vi "Teleop.vi"(10 "Match Info":T2={"Autonomous Elapsed Seconds"=0.0, "TeleOp Elapsed Seconds"=0.0, "Disabled Elapsed Seconds"=0.0, "Visited Autonomous"=FALSE, "Visited TeleOp"=FALSE, "Visited Disabled"=FALSE, "Autonomous Settings"={"Autonomous Style"=enum."Independent", "VI Refnum"=refnum}}, 11 "Call Context":T3) -> ()   [LabVIEW 2019]
doc: "This VI is called for each TeleOp packet received from the DS where the robot is not disabled. It is often used to read from the joysticks and update I/O or to update setpoints for timed control loops. It should complete and return within 20 milliseconds or it may miss DS packets."
uses:
  <vilib>/Rock Robotics/WPI/DriverStation/WPI_DriverStationDerivedRobotMode.ctl
  <vilib>/Rock Robotics/WPI/DriverStation/WPI_DriverStationMatch Info.ctl
  <vilib>/Rock Robotics/WPI/Utilities/WPI_GetSetVariantRefNum.vi
  <vilib>/Rock Robotics/Network Tables/NT Write Boolean Array.vi
  <vilib>/Rock Robotics/Network Tables/NT Write Numeric Array.vi
  <vilib>/Rock Robotics/Network Tables/NT Read Boolean.vi
  <vilib>/Rock Robotics/Network Tables/NT Read Number.vi
  <vilib>/Rock Robotics/Network Tables/NT Write Number.vi
  <vilib>/Rock Robotics/WPI/RobotDrive/WPI_RobotDriveMecanumDrive_Cartesian.vi
  <vilib>/Instr/_visa.llb/VISA Configure Serial Port (Instr).vi
  <vilib>/Rock Robotics/Network Tables/NT Write String.vi
panel:
  out "read buffer":string="0"
  out "return count":u32
  out "Continuous Angle":T1
  out "x":i16
  out "Matched Color Name":string
  out "Match Confidence":dbl
  out "Measured Color":cluster{"R":dbl, "G":dbl, "B":dbl}
  out "error out":errorcluster
  out "Color":u32(colorbox)
  in  "Blue Calibration":cluster{"R":dbl, "G":dbl, "B":dbl}={"R"=0.143, "G"=0.427, "B"=0.429}
  in  "Green Calibration":cluster{"R":dbl, "G":dbl, "B":dbl}={"R"=0.197, "G"=0.561, "B"=0.24}
  in  "Red Calibration":cluster{"R":dbl, "G":dbl, "B":dbl}={"R"=0.561, "G"=0.323, "B"=0.114}
  in  "Yellow Calibration":cluster{"R":dbl, "G":dbl, "B":dbl}={"R"=0.361, "G"=0.524, "B"=0.113}
  out "Elapsed Time Since Reset (s)":i32 caption="Elapsed Time (s)"
  out "Sample Slider 0":dbl(slide) scale=0.0..5.0
  out "Sample Boolean 1":bool
  out "Sample Boolean 0":bool
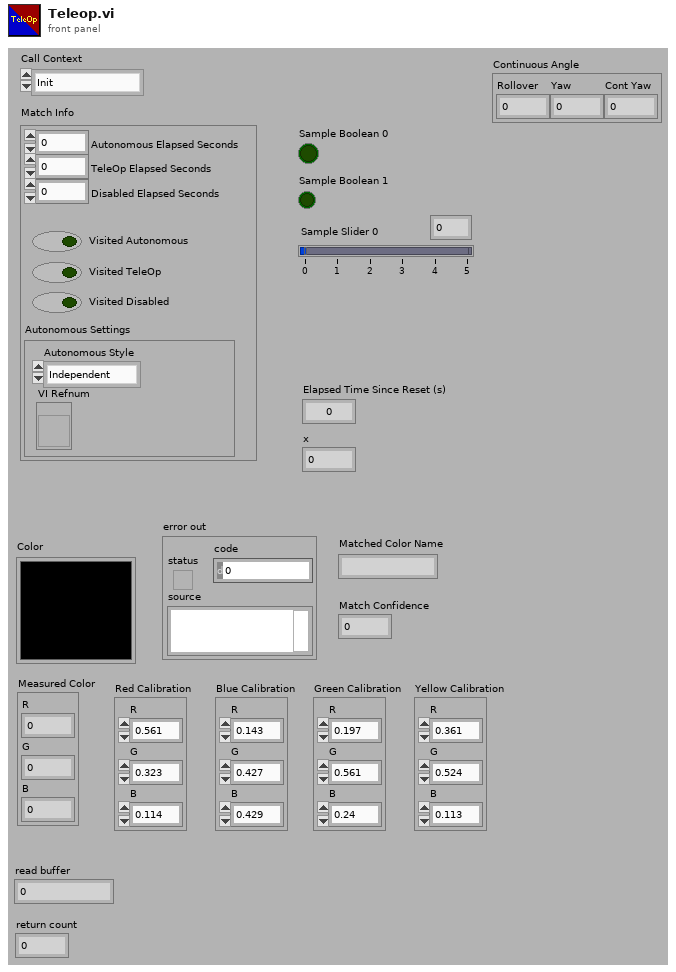
[diagram p1: front panel]
types:
  T1 = cluster{"Rollover":dbl, "Yaw":dbl, "Cont Yaw":dbl}
  T2 = typedef "WPI_DriverStationMatch Info.ctl" = cluster{"Autonomous Elapsed Seconds":dbl, "TeleOp Elapsed Seconds":dbl, "Disabled Elapsed Seconds":dbl, "Visited Autonomous":bool, "Visited TeleOp":bool, "Visited Disabled":bool, "Autonomous Settings":cluster{"Autonomous Style":enum16{"Iterative", "Independent"}, "VI Refnum":refnum<vi>}}
  T3 = typedef "WPI_DriverStationDerivedRobotMode.ctl" = enum16{"Init", "Execute", "Stop"}
  T4 = typedef "Color Sensor V3 DevRef.ctl" = cluster{"I2CDevRef":T5}
  T5 = typedef "WPI_I2CDevRef.ctl" = cluster{"DevStatus":errorcluster, "Device Address":u8, "Handle":i32, "I2C Bus":T6}
  T6 = typedef "i2c_bus.ctl" = enum16{"I2C On-Board", "I2C MXP", "Invalid"}
  T7 = typedef "WPI_RobotDriveDevRef.ctl" = cluster{"DevStatus":errorcluster, "Motors[]":T8[], "Square Inputs":bool, "Max Output":dbl}
  T8 = typedef "WPI_MotorControlDeviceRef.ctl" = cluster{"DeviceStatus":errorcluster, "Type":T9, "PWM":cluster{"PWM Channel":T10, "DeadBand":T11}, "CAN":cluster{"Device Number":u8, "SetOutput VI Ref":variant, "GetOutput VI Ref":variant, "Enable VI Ref":variant, "Disable VI Ref":variant, "Data":variant}, "Invert":bool, "DIO PWM":cluster{"PWM \"Enable\" Channel":T10, "DIOChannel":T12, "PWM Rate":dbl}}
  T9 = typedef "WPI_MotorControlType.ctl" = enum16{"PWM", "CAN", "DIO PWM"}
  T10 = typedef "FPGA_DIOPWMChannel.ctl" = enum8{"PWM 0", "PWM 1", "PWM 2", "PWM 3", "PWM 4", "PWM 5", "PWM 6", "PWM 7", "PWM 8", "PWM 9", "PWM MXP 0", "PWM MXP 1", "PWM MXP 2", "PWM MXP 3", "PWM MXP 4", "PWM MXP 5", "PWM MXP 6", "PWM MXP 7", "PWM MXP 8", "PWM MXP 9", "Invalid"}
  T11 = typedef "WPI_PWMDeadband.ctl" = cluster{"Name":string, "maxPositivePwm":i32, "minPositivePwm":i32, "centerPwm":i32, "maxNegativePwm":i32, "minNegativePwm":i32, "angularRange":u16}
  T12 = typedef "FPGA_DIOChannel.ctl" = enum8{"DIO 0", "DIO 1", "DIO 2", "DIO 3", "DIO 4", "DIO 5", "DIO 6", "DIO 7", "DIO 8", "DIO 9", "DIO MXP 0", "DIO MXP 1", "DIO MXP 2", "DIO MXP 3", "DIO MXP 4", "DIO MXP 5", "DIO MXP 6", "DIO MXP 7", "DIO MXP 8", "DIO MXP 9", "DIO MXP 10", "DIO MXP 11", "DIO MXP 12", "DIO MXP 13", "DIO MXP 14", "DIO MXP 15", "SPI Port CS1", "SPI Port CS2", "SPI Port CS3", "SPI Port MISO", "SPI Port MOSI", "Invalid"}
  T13 = typedef "WPI_JoystickDevRef.ctl" = cluster{"Device":T14}
  T14 = typedef "WPI_JoystickDeviceEnum.ctl" = enum16{"USB 0", "USB 1", "USB 2", "USB 3", "USB 4", "USB 5"}
  T15 = typedef "WPI_SwitchDevRef.ctl" = cluster{"DevStatus":errorcluster, "DIO Channel":T12, "CntIndex":T16, "Normally Closed":bool}
  T16 = typedef "FPGA_CounterCtrSystemIndex.ctl" = enum8{"Ctr 0", "Ctr 1", "Ctr 2", "Ctr 3", "Ctr 4", "Ctr 5", "Ctr 6", "Ctr 7", "Invalid"}
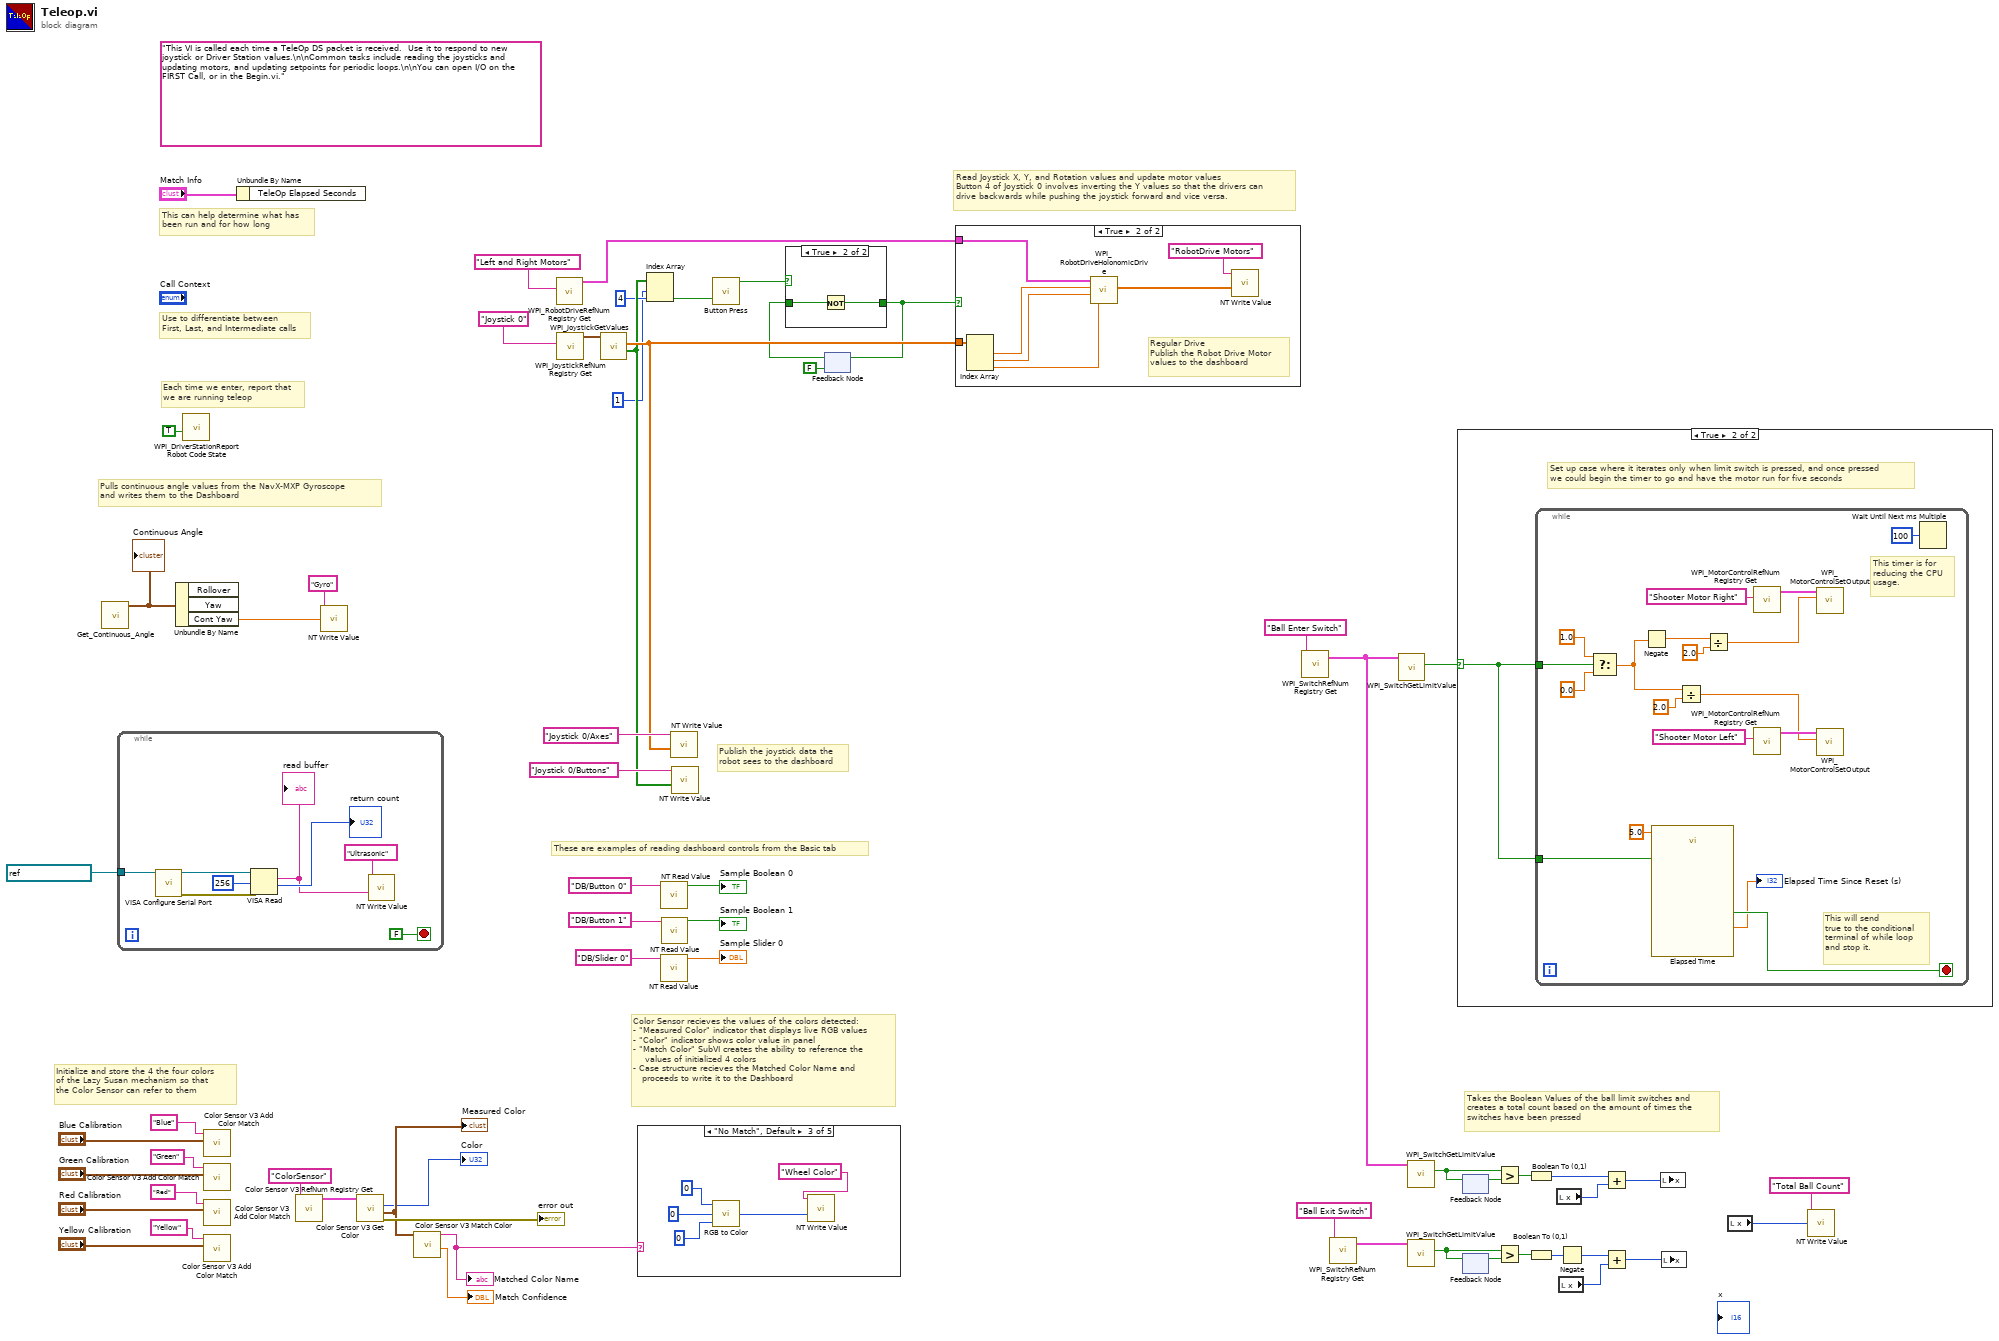
[diagram p0: block diagram]
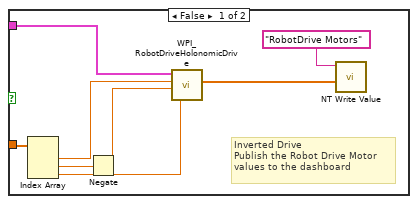
[diagram p2: hidden frame]
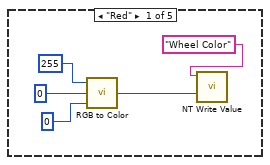
[diagram p4: hidden frame]
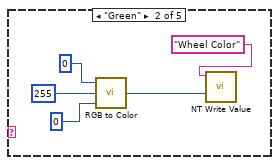
[diagram p5: hidden frame]
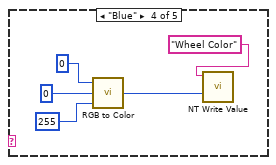
[diagram p6: hidden frame]
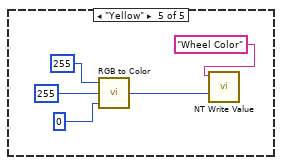
[diagram p7: hidden frame]
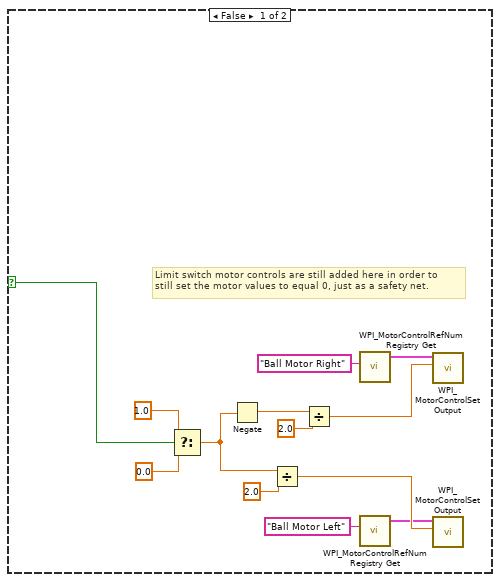
[diagram p8: hidden frame]
diagram:
  (unwired) "This VI is called each time a TeleOp DS packet is received.  Use it to respond to new joystick or Driver Station values.\n\nCommon tasks include reading the joysticks and updating motors, and updating setpoints for periodic loops.\n\nYou can open I/O on the FIRST Call, or in the Begin.vi."
  # "Takes the Boolean Values of the ball limit switches and \ncreates a total count based on the amount of times the \nswitches have been pressed"
  # "Pulls continuous angle values from the NavX-MXP Gyroscope\nand writes them to the Dashboard"
  # "Color Sensor recieves the values of the colors detected:\n- \"Measured Color\" indicator that displays live RGB values\n- \"Color\" indicator shows color value in panel\n- \"Match Color\" SubVI creates the ability to reference the \n    values of initialized 4 colors\n- Case structure recieves the Matched Color Name and \n   proceeds to write it to the Dashboard"
  # "Initialize and store the 4 the four colors \nof the Lazy Susan mechanism so that \nthe Color Sensor can refer to them"
  # "These are examples of reading dashboard controls from the Basic tab"
  # "Publish the joystick data the\nrobot sees to the dashboard"
  # "Each time we enter, report that\nwe are running teleop"
  # "Use to differentiate between\nFirst, Last, and Intermediate calls"
  # "This can help determine what has\nbeen run and for how long"
  # "Read Joystick X, Y, and Rotation values and update motor values\nButton 4 of Joystick 0 involves inverting the Y values so that the drivers can\ndrive backwards while pushing the joystick forward and vice versa."
  n1 = call <vilib>:"Get_Continuous_Angle.vi"() -> ("Continuous Angle"=w2:T1)  [unwired: 11 in]
  "Continuous Angle" <- w2
  n2 = while {
    tunnel: refnum<visa-resource-name> "ASRL3::INSTR" ("VISA resource name") -> [w66]
    stop <- FALSE stop-if-true
    n3 = call-poly "VISA Configure Serial Port"("VISA resource name"=w66) -> ("VISA resource name out"=w70:refnum<visa-resource-name>, "error out"=w68:errorcluster)  [unwired: 13 in]
    n4 = VISA Read(VISA resource name=w70, byte count=u32 256, error in (no error)=w68) -> (read buffer=w63:string, return count=→"return count":u32)  [unwired: 2 out]
    "read buffer" <- w63
    n5 = call-poly <vilib>:"NT Write Value.vi"("String"=w63, "Name"="Ultrasonic") -> ()  [unwired: 9 in, 1 out]
  }
  n6 = Unbundle By Name(w2) -> ("Cont Yaw"=w4:dbl)  [unwired: 2 out]
  n7 = call <vilib>:"WPI_DriverStationReport Robot Code State.vi"("TeleOp"=TRUE ("Autonomous")) -> ()  [unwired: 10 in, 1 out]
  n8 = call <vilib>:"Color Sensor V3 Add Color Match.vi"("Color"="Blue Calibration", "Name"="Blue") -> ()  [unwired: 10 in]
  n9 = call <vilib>:"Color Sensor V3 Add Color Match.vi"("Color"="Green Calibration", "Name"="Green") -> ()  [unwired: 10 in]
  n10 = call <vilib>:"Color Sensor V3 Add Color Match.vi"("Color"="Red Calibration", "Name"="Red") -> ()  [unwired: 10 in]
  n11 = call <vilib>:"Color Sensor V3 Add Color Match.vi"("Color"="Yellow Calibration", "Name"="Yellow") -> ()  [unwired: 10 in]
  n12 = Unbundle By Name("Match Info") -> ()  [unwired: 1 out]
  n13 = call <vilib>:"Color Sensor V3 RefNum Registry Get.vi"("refnum name"="ColorSensor") -> ("ColorSensorDevRef"=w32:T4)  [unwired: 9 in, 1 out]
  n14 = call-poly <vilib>:"NT Write Value.vi"("Numeric"=w4, "Name"="Gyro") -> ()  [unwired: 9 in, 1 out]
  n15 = call <vilib>:"Color Sensor V3 Get Color.vi"("ColorSensorDevRef"=w32) -> ("error out"=→"error out":errorcluster, "Normalized Color"=w34:cluster{"R":dbl, "G":dbl, "B":dbl}, "Color"=→"Color":u32)  [unwired: 7 in, 1 out]
  "Measured Color" <- w34
  n16 = call <vilib>:"Color Sensor V3 Match Color.vi"("Measured Color"=w34) -> ("Confidence"=→"Match Confidence":dbl, "Matched Color Name"=w21:string)  [unwired: 8 in, 1 out]
  "Matched Color Name" <- w21
  n17 = call <vilib>:"WPI_RobotDriveRefNum Registry Get.vi"("refnum name"="Left and Right Motors") -> ("RobotDriveDevRef"=w22:T7)  [unwired: 1 in, 9 out]
  n18 = call <vilib>:"WPI_JoystickRefNum Registry Get.vi"("refnum name"="Joystick 0") -> ("JoystickDevRef"=w59:T13)  [unwired: 1 in, 9 out]
  n19 = call <vilib>:"WPI_JoystickGetValues.vi"("JoystickDevRef"=w59) -> ("Buttons"=w20:bool[], "Axes"=w55:dbl[])  [unwired: 6 in, 3 out]
  n20 = case shown="\"No Match\", Default" w21 {
    frame "Red" {
      n21 = call <vilib>:"RGB to Color.vi"("B"=u8 0, "G"=u8 0, "R"=u8 255) -> ("Color"=w71:u32)
      n22 = call-poly <vilib>:"NT Write Value.vi"("Numeric"=w71, "Name"="Wheel Color") -> ()  [unwired: 9 in, 1 out]
    }
    frame "Green" {
      n23 = call <vilib>:"RGB to Color.vi"("B"=u8 0, "G"=u8 255, "R"=u8 0) -> ("Color"=w76:u32)
      n24 = call-poly <vilib>:"NT Write Value.vi"("Numeric"=w76, "Name"="Wheel Color") -> ()  [unwired: 9 in, 1 out]
    }
    frame "No Match", Default {
      n25 = call <vilib>:"RGB to Color.vi"("B"=u8 0, "G"=u8 0, "R"=u8 0) -> ("Color"=w81:u32)
      n26 = call-poly <vilib>:"NT Write Value.vi"("Numeric"=w81, "Name"="Wheel Color") -> ()  [unwired: 9 in, 1 out]
    }
    frame "Blue" {
      n27 = call <vilib>:"RGB to Color.vi"("B"=u8 255, "G"=u8 0, "R"=u8 0) -> ("Color"=w86:u32)
      n28 = call-poly <vilib>:"NT Write Value.vi"("Numeric"=w86, "Name"="Wheel Color") -> ()  [unwired: 9 in, 1 out]
    }
    frame "Yellow" {
      n29 = call <vilib>:"RGB to Color.vi"("B"=u8 0, "G"=u8 255, "R"=u8 255) -> ("Color"=w95:u32)
      n30 = call-poly <vilib>:"NT Write Value.vi"("Numeric"=w95, "Name"="Wheel Color") -> ()  [unwired: 9 in, 1 out]
    }
  }
  n31 = Index Array(array=w20, index #1=1 ("index"), index #2=4 ("index")) -> (element #2=w19:bool)  [unwired: 1 out]
  n32 = call-poly <vilib>:"NT Read Value.vi"("Name"="DB/Button 0" ("refnum name")) -> ("Boolean"=→"Sample Boolean 0":bool)  [unwired: 9 in, 1 out]
  n33 = call-poly <vilib>:"NT Read Value.vi"("Name"="DB/Slider 0" ("refnum name")) -> ("Numeric"=→"Sample Slider 0":dbl)  [unwired: 9 in, 1 out]
  n34 = call-poly <vilib>:"NT Read Value.vi"("Name"="DB/Button 1" ("refnum name")) -> ("Boolean"=→"Sample Boolean 1":bool)  [unwired: 9 in, 1 out]
  n35 = call-poly <vilib>:"NT Write Value.vi"("Numeric Array"=w55, "Name"="Joystick 0/Axes") -> ()  [unwired: 9 in, 1 out]
  n36 = call-poly <vilib>:"NT Write Value.vi"("Boolean Array"=w20, "Name"="Joystick 0/Buttons") -> ()  [unwired: 9 in, 1 out]
  n37 = call "Button Press.vi"("Button In"=w19) -> ("Button Pressed?"=w18:bool)  [unwired: 10 in]
  n38 = feedback #1(FALSE) -> (w17:bool)
  n39 = case shown="True" w18 {
    tunnel: w17 -> [w96 w98]
    tunnel: [w96 w97] -> w15
    frame False {
    }
    frame True {
      n40 = Not(x=w98) -> (.not. x?=w97:bool)
    }
  }
  n41 = feedback-in #1(w15) -> ()
  n42 = case shown="True" w15 {
    tunnel: w55 -> [w101 w113]
    tunnel: w22 -> [w102 w109]
    frame False {
      # "Inverted Drive\nPublish the Robot Drive Motor\nvalues to the dashboard"
      n43 = Index Array(array=w101) -> (element #1=w104:dbl, element #2=w100:dbl, element #3=w106:dbl)  [unwired: 3 in]
      n44 = Negate(x=w100) -> (-x=w99:dbl)
      n45 = call-poly <vilib>:"WPI_RobotDriveHolonomicDrive.vi"("Rotation"=w106, "Y"=w99, "X"=w104, "RobotDriveDevRef"=w102) -> ("Motor Values"=w105:dbl[])  [unwired: 5 in, 2 out]
      n46 = call-poly <vilib>:"NT Write Value.vi"("Numeric Array"=w105, "Name"="RobotDrive Motors") -> ()  [unwired: 9 in, 1 out]
    }
    frame True {
      # "Regular Drive\nPublish the Robot Drive Motor\nvalues to the dashboard"
      n47 = Index Array(array=w113) -> (element #1=w110:dbl, element #2=w111:dbl, element #3=w107:dbl)  [unwired: 3 in]
      n48 = call-poly <vilib>:"WPI_RobotDriveHolonomicDrive.vi"("Rotation"=w107, "Y"=w111, "X"=w110, "RobotDriveDevRef"=w109) -> ("Motor Values"=w108:dbl[])  [unwired: 5 in, 2 out]
      n49 = call-poly <vilib>:"NT Write Value.vi"("Numeric Array"=w108, "Name"="RobotDrive Motors") -> ()  [unwired: 9 in, 1 out]
    }
  }
  n50 = call <vilib>:"WPI_SwitchRefNum Registry Get.vi"("refnum name"="Ball Enter Switch") -> ("SwitchDevRef"=w13:T15)  [unwired: 9 in, 1 out]
  n51 = call <vilib>:"WPI_SwitchRefNum Registry Get.vi"("refnum name"="Ball Exit Switch") -> ("SwitchDevRef"=w23:T15)  [unwired: 9 in, 1 out]
  n52 = call <vilib>:"WPI_SwitchGetLimitValue.vi"("SwitchDevRef"=w13) -> ("Switch Pressed"=w47:bool)  [unwired: 8 in, 2 out]
  n53 = call <vilib>:"WPI_SwitchGetLimitValue.vi"("SwitchDevRef"=w13) -> ("Switch Pressed"=w24:bool)  [unwired: 8 in, 2 out]
  n54 = call <vilib>:"WPI_SwitchGetLimitValue.vi"("SwitchDevRef"=w23) -> ("Switch Pressed"=w27:bool)  [unwired: 8 in, 2 out]
  n55 = case shown="True" w47 {
    selector: w47 -> [w114 w127]
    frame False {
      # "Limit switch motor controls are still added here in order to \nstill set the motor values to equal 0, just as a safety net."
      n56 = Select(t=1.0, s=w114, f=0.0) -> (s? t:f=w123:dbl)
      n57 = Negate(x=w123) -> (-x=w125:dbl)
      n58 = Divide(x=w123, y=2.0) -> (x/y=w124:dbl)
      n59 = Divide(x=w125, y=2.0) -> (x/y=w126:dbl)
      n60 = call <vilib>:"WPI_MotorControlRefNum Registry Get.vi"("refnum name"="Ball Motor Right") -> ("MotorControlDevRef"=w122:T8)  [unwired: 9 in, 1 out]
      n61 = call <vilib>:"WPI_MotorControlRefNum Registry Get.vi"("refnum name"="Ball Motor Left") -> ("MotorControlDevRef"=w121:T8)  [unwired: 9 in, 1 out]
      n62 = call <vilib>:"WPI_MotorControlSetOutput.vi"("Output"=w126, "MotorControlDevRef"=w122) -> ()  [unwired: 7 in, 3 out]
      n63 = call <vilib>:"WPI_MotorControlSetOutput.vi"("Output"=w124, "MotorControlDevRef"=w121) -> ()  [unwired: 7 in, 3 out]
    }
    frame True {
      # "Set up case where it iterates only when limit switch is pressed, and once pressed \nwe could begin the timer to go and have the motor run for five seconds"
      n64 = while {
        tunnel: w127 -> [w128]
        tunnel: w127 -> [w129]
        stop <- w145 stop-if-true
        # "This timer is for\nreducing the CPU\nusage."
        # "This will send\ntrue to the conditional\nterminal of while loop \nand stop it."
        n65 = Select(t=1.0, s=w129, f=0.0) -> (s? t:f=w135:dbl)
        n66 = Negate(x=w135) -> (-x=w132:dbl)
        n67 = call "Elapsed Time"("Time Target (s)"=5.0, "Auto Reset"=w128) -> ("Elapsed Time (s)"=→"Elapsed Time Since Reset (s)":dbl, "Time has Elapsed"=w145:bool)  [unwired: 10 in, 6 out]
        n68 = Divide(x=w135, y=2.0) -> (x/y=w133:dbl)
        n69 = Divide(x=w132, y=2.0) -> (x/y=w130:dbl)
        n70 = call <vilib>:"WPI_MotorControlRefNum Registry Get.vi"("refnum name"="Shooter Motor Right") -> ("MotorControlDevRef"=w137:T8)  [unwired: 9 in, 1 out]
        n71 = call <vilib>:"WPI_MotorControlRefNum Registry Get.vi"("refnum name"="Shooter Motor Left") -> ("MotorControlDevRef"=w141:T8)  [unwired: 9 in, 1 out]
        n72 = call <vilib>:"WPI_MotorControlSetOutput.vi"("Output"=w130, "MotorControlDevRef"=w137) -> ()  [unwired: 7 in, 3 out]
        n73 = call <vilib>:"WPI_MotorControlSetOutput.vi"("Output"=w133, "MotorControlDevRef"=w141) -> ()  [unwired: 7 in, 3 out]
        n74 = Wait Until Next ms Multiple(millisecond multiple=u32 100) -> ()  [unwired: 1 out]
      }
    }
  }
  n75 = feedback #2() -> (w25:bool)  [unwired: 1 in]
  n76 = feedback-in #2(w24) -> ()
  n77 = feedback #3() -> (w28:bool)  [unwired: 1 in]
  n78 = feedback-in #3(w27) -> ()
  n79 = Greater?(x=w24, y=w25) -> (0:w26:bool)
  n80 = Greater?(x=w27, y=w28) -> (0:w29:bool)
  n81 = Boolean To (0,1)(Boolean=w26) -> (0, 1=w9:i16)
  n82 = Boolean To (0,1)(Boolean=w29) -> (0, 1=w30:i16)
  n83 = local read "x"() -> (w8:i16)
  n84 = Negate(x=w30) -> (-x=w12:i16)
  n85 = local read "x"() -> (w11:i16)
  n86 = Add(x=w9, y=w8) -> (x+y=w7:i16)
  n87 = Add(x=w12, y=w11) -> (x+y=w10:i16)
  n88 = local write "x"(w7) -> ()
  n89 = local write "x"(w10) -> ()
  n90 = local read "x"() -> (w6:i16)
  n91 = call-poly <vilib>:"NT Write Value.vi"("Numeric"=w6, "Name"="Total Ball Count") -> ()  [unwired: 9 in, 1 out]
